vi "get_shutter.vi"(8 "error in (no error)":errorcluster, 11 "LightSourceScaffold in":refnum<class "LightSourceScaffold.lvclass">) -> (0 "error out":errorcluster, 2 "shutter open out?":bool, 3 "LightSourceScaffold out":refnum<class "LightSourceScaffold.lvclass">)   [LabVIEW 2010, in "LightSourceScaffold.lvclass"]
uses:
  LightSourceScaffold.lvclass
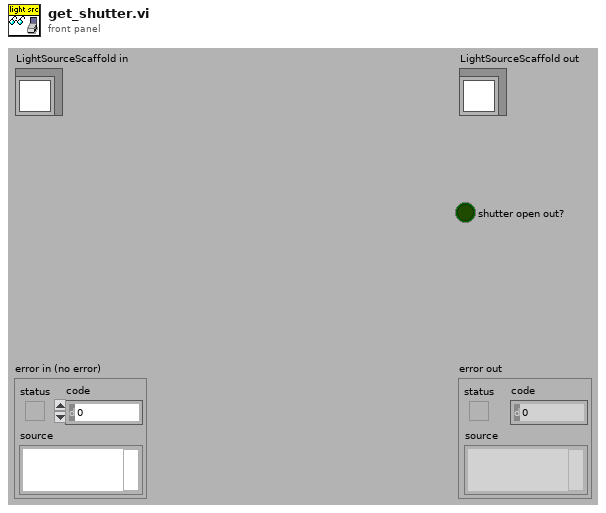
[diagram p1: front panel]
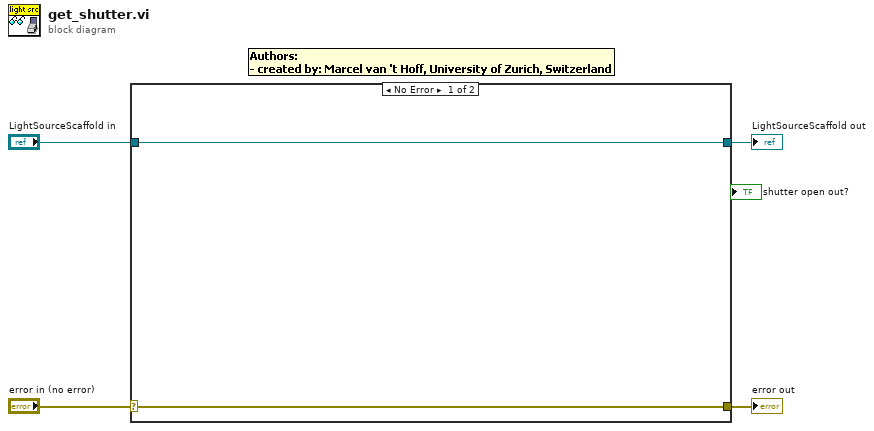
[diagram p0: block diagram]
diagram:
  n1 = case shown="No Error" "error in (no error)" {
    selector: "error in (no error)" -> [w5 w8]
    tunnel: [w5 w8] -> w3
    tunnel: [w6 w7] -> w1
    tunnel: "LightSourceScaffold in" -> [w6 w7]
    frame No Error {
    }
    frame Error {
    }
  }
  "error out" <- w3
  "LightSourceScaffold out" <- w1
